vi "setSerializedData.vi"(0 "reference in":refnum<class "VINode.lvclass">, 1 "parent":refnum<class "AbstractNode.lvclass">, 2 "children":refnum<class "AbstractNode.lvclass">[](array[class]), 3 "xmlIn":string, 5 "error in (no error)":errorcluster) -> (14 "reference out":refnum<class "VINode.lvclass">, 19 "error out":errorcluster)   [LabVIEW 2014, in "VINode.lvclass"]
doc: "Sets stored data"
uses:
  <resource>/Framework/Providers/Open_GDS/UML/VINode_class/VINode.lvclass
  <resource>/Framework/Providers/Open_GDS/UML/AbstractNode_class/AbstractNode.lvclass
  <resource>/Framework/Providers/Open_GDS/UML/AbstractNode_class/protected/ObjectAttributes.ctl
  <resource>/Framework/Providers/Open_GDS/UML/RectangularNode_class/protected/ObjectAttributes.ctl
  <resource>/Framework/Providers/Open_GDS/UML/General/Rectangle/Rectangle Rectangle2D.ctl
  <resource>/Framework/Providers/Open_GDS/UML/VINode_class/protected/ObjectAttributes.ctl
  <resource>/Framework/Providers/Open_GDS/UML/MultiLineString_class/MultiLineString.lvclass
  <resource>/Framework/Providers/Open_GDS/UML/RectangularNode_class/RectangularNode.lvclass
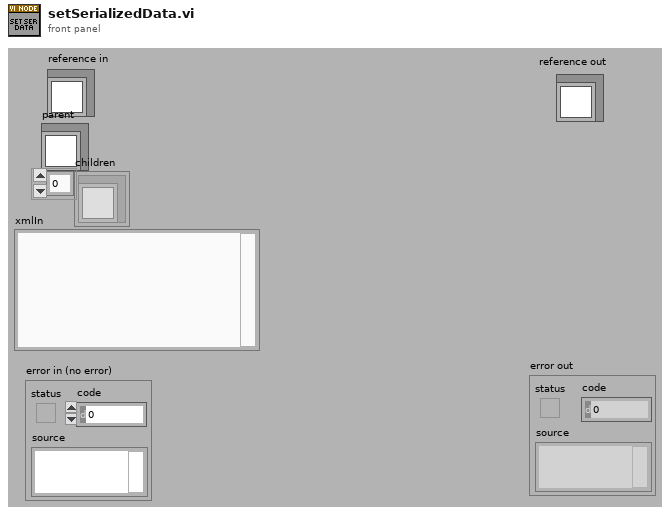
[diagram p1: front panel]
types:
  T1 = cluster{"data string":string, "text":string, "text 2":string}
  T2 = typedef "AbstractNode.lvclass/ObjectAttributes.ctl" = cluster{"parent":refnum<class "AbstractNode.lvclass">, "children":refnum<class "AbstractNode.lvclass">[], "Hidden":bool}
  T3 = typedef "RectangularNode.lvclass/ObjectAttributes.ctl" = cluster{"bounds":T4}
  T4 = typedef "Rectangle Rectangle2D.ctl" = cluster{"x":dbl, "y":dbl, "width":dbl, "height":dbl}
  T5 = typedef "VINode.lvclass/ObjectAttributes.ctl" = cluster{"midHeight":dbl, "botHeight":dbl, "Name":refnum<class "MultiLineString.lvclass">, "DEFAULT_COMPARTMENT_HEIGHT":i32, "DEFAULT_WIDTH":i32, "DEFAULT_HEIGHT":i32, "ClassPath":path, "Icon":u8[][], "Description":refnum<class "MultiLineString.lvclass">, "ShowDescription":bool}
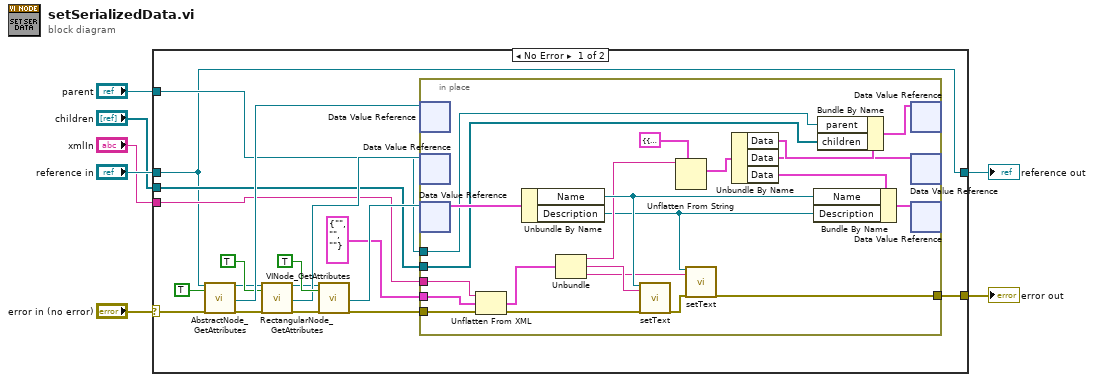
[diagram p0: block diagram]
diagram:
  n1 = case shown="No Error" "error in (no error)" {
    selector: "error in (no error)" -> [w16 w48]
    tunnel: "reference in" -> [w9 w49]
    tunnel: [w25 w48] -> w5
    tunnel: [w9 w49] -> w4
    tunnel: "xmlIn" -> [w20 _]
    tunnel: "parent" -> [w19 _]
    tunnel: "children" -> [w18 _]
    frame No Error {
      n2 = call <resource>:"AbstractNode_GetAttributes.vi"("reference in"=w9, "OnlyGetDvrReference(False)"=TRUE, "error in (no error)"=w16) -> ("reference out"=w13:refnum<class "VINode.lvclass">, "DataRef"=w21:refnum<data-value>, "error out"=w14:errorcluster)  [unwired: 13 in, 1 out]
      n3 = call <resource>:"RectangularNode_GetAttributes.vi"("reference in"=w13, "OnlyGetDvrReference(False)"=TRUE, "error in (no error)"=w14) -> ("reference out"=w12:refnum<class "VINode.lvclass">, "DataRef"=w22:refnum<data-value>, "error out"=w11:errorcluster)  [unwired: 13 in, 1 out]
      n4 = call <resource>:"VINode_GetAttributes.vi"("reference in"=w12, "OnlyGetDvrReference(False)"=TRUE, "error in (no error)"=w11) -> ("DataRef"=w23:refnum<data-value>, "error out"=w10:errorcluster)  [unwired: 13 in, 2 out]
      n5 = in-place {
        in-place-border: [w26] -> w25
        in-place-border: w10 -> [w34]
        in-place-border: T1 {"data string"="", "text"="", "text 2"=""} ("output cluster") -> [w46]
        in-place-border: w20 -> [w47]
        in-place-border: w19 -> [w36]
        in-place-border: w18 -> [w35]
        n6 = in-place-dvr #1(w21) -> ()  [unwired: 2 out]
        n7 = in-place-dvr #2(w22) -> ()  [unwired: 2 out]
        n8 = in-place-dvr #3(w23) -> (w40:T5)  [unwired: 1 out]
        n9 = Unflatten From XML(xml string=w47, type=w46, error in (no error)=w34) -> (value=w45:T1, error out=w33:errorcluster)
        n10 = Unbundle By Name(w40) -> ("Name"=w39:refnum<class "MultiLineString.lvclass">, "Description"=w29:refnum<class "MultiLineString.lvclass">)
        n11 = Unbundle(w45) -> ("data string"=w32:string, "text"=w38:string, "text 2"=w28:string)
        n12 = call-dynamic "setText.vi"("reference"=w39, "text"=w38, "error in (no error)"=w33) -> ("error out"=w27:errorcluster)  [unwired: 15 in, 1 out]
        n13 = Unflatten From String(type=cluster{"Data":T2, "Data":T3, "Data":T5} {"Data"={"parent"=refnum, "children"=[], "Hidden"=FALSE}, "Data"={"bounds"={"x"=0.0, "y"=0.0, "width"=0.0, "height"=0.0}}, "Data"={"midHeight"=0.0, "botHeight"=0.0, "Name"=refnum, "DEFAULT_COMPARTMENT_HEIGHT"=0, "DEFAULT_WIDTH"=0, "DEFAULT_HEIGHT"=0, "ClassPath"=path "", "Icon"=[], "Description"=refnum, "ShowDescription"=FALSE}}, binary string=w32) -> (value=w30:cluster{"Data":T2, "Data":T3, "Data":T5})  [unwired: 3 in, 2 out]
        n14 = call-dynamic "setText.vi"("reference"=w29, "text"=w28, "error in (no error)"=w27) -> ("error out"=w26:errorcluster)  [unwired: 15 in, 1 out]
        n15 = Unbundle By Name(w30) -> ("Data"=w44:T2, "Data"=w43:T3, "Data"=w42:T5)
        n16 = Bundle By Name(cluster=w42, "Name"=w39, "Description"=w29) -> (w41:T5)
        n17 = Bundle By Name(cluster=w44, "parent"=w36, "children"=w35) -> (w37:T2)
        n18 = in-place-dvr #1(w37) -> ()  [unwired: 2 out]
        n19 = in-place-dvr #2(w43) -> ()  [unwired: 2 out]
        n20 = in-place-dvr #3(w41) -> ()  [unwired: 2 out]
      }
    }
    frame Error {
    }
  }
  "reference out" <- w4
  "error out" <- w5
